vi "V_to_I16Dim.vi"(8 "Max/Min Value [V]":dbl, 11 "Input":dbl[](array[numeric])=[0.0, 0.0]) -> (2 "16bit integer":i16[](array[numeric]))   [LabVIEW 2023]
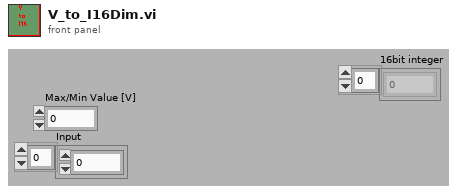
[diagram p1: front panel]
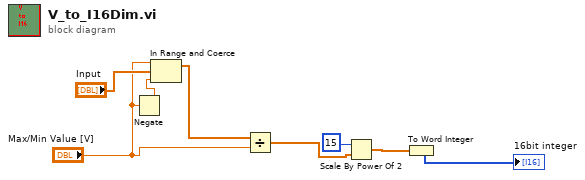
[diagram p0: block diagram]
diagram:
  n1 = Negate(x="Max/Min Value [V]") -> (-x=w2:dbl)
  n2 = In Range and Coerce(upper limit="Max/Min Value [V]", x="Input", lower limit=w2) -> (coerced(x)=w1:dbl[])  [unwired: 1 out]
  n3 = Divide(x=w1, y="Max/Min Value [V]") -> (x/y=w7:dbl[])
  n4 = Scale By Power Of 2(n=15, x=w7) -> (x*2^n=w6:dbl[])
  n5 = To Word Integer(number=w6) -> (16bit integer=→"16bit integer":i16[])
